vi "Copy Array to Image (Pixels).vi"(8 "error in (no error)":errorcluster, 10 "ARGB Image Destination in":T1, 11 "(A)RGB Pixels Data":u8[][][](array[numeric])) -> (0 "error out":errorcluster, 3 "ARGB Image Destination":T1)   [LabVIEW 2020, in "image.lvlib"]
doc: "Copy a 3D array of (A)RGB pixel data into the Destination Image. The Destination Image will be resized to fit the Array Data."
uses:
  image.lvlib
  ARGB Image.ctl
  common/common.lvlib
  common/bin/gartoolkit_32-1.dll
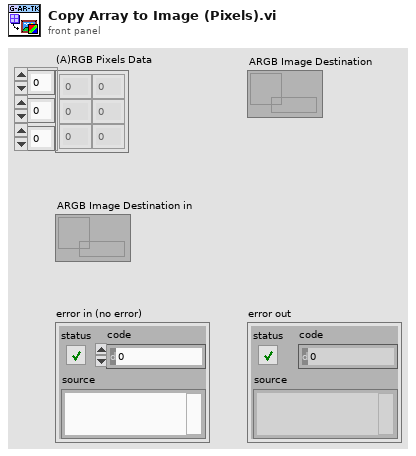
[diagram p1: front panel]
types:
  T1 = typedef "image.lvlib/ARGB Image.ctl" = refnum<data-value>
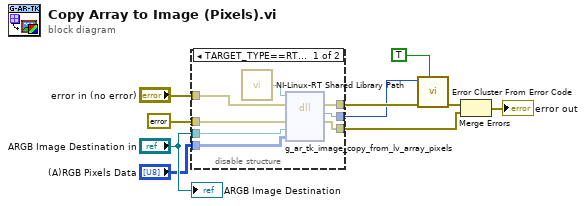
[diagram p0: block diagram]
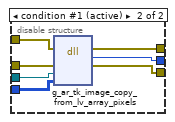
[diagram p2: hidden frame]
diagram:
  n1 = disable-structure shown="TARGET_TYPE==RT&&OS==Linux" {
    disable-tunnel: "error in (no error)" -> [w18 w25]
    disable-tunnel: errorcluster {"status"=FALSE, "code"=0, "source"=""} ("error constant") -> [w17 w24]
    disable-tunnel: "ARGB Image Destination in" -> [w16 w23]
    disable-tunnel: "(A)RGB Pixels Data" -> [w15 w22]
    disable-tunnel: [w14 w21] -> w4
    disable-tunnel: [w13 w20] -> w3
    disable-tunnel: [w12 w19] -> w2
    frame condition #0 {
      n2 = call "NI-Linux-RT Shared Library Path.vi"() -> ("Path"=w11:path)
      n3 = dll-call lib="?" fn="g_ar_tk_image_copy_from_lv_array_pixels" ("g_ar_toolkit.*.*:g_ar_tk_image_copy_from_raw_memory")(path in=w11, error in=w18, "error_cluster"=w17, "edvr_dst"=w16, "array"=w15) -> (error out=w14:errorcluster, w13:i32, "error_cluster"=w12:errorcluster)  [unwired: 3 in, 1 out]
    }
    frame condition #1 (active) {
      n4 = dll-call lib="C:/serenial/lib/g-augmented-reality-toolkit/LabVIEW/common/bin/gartoolkit_*-1.*" fn="g_ar_tk_image_copy_from_lv_array_pixels" ("g_ar_toolkit.*.*:g_ar_tk_image_copy_from_raw_memory")(error in=w25, "error_cluster"=w24, "edvr_dst"=w23, "array"=w22) -> (error out=w21:errorcluster, w20:i32, "error_cluster"=w19:errorcluster)  [unwired: 4 in, 1 out]
    }
  }
  n5 = call <vilib>:"Error Cluster From Error Code.vi"("show call chain? (False)"=TRUE, "error in (no error)"=w4, "error code (0)"=w3) -> ("error out"=w9:errorcluster)  [unwired: 6 in]
  n6 = Merge Errors(w9, w2) -> (→"error out":errorcluster)
  "ARGB Image Destination" <- "ARGB Image Destination in"
